vi "Get Pumpstage.vi"(8 "error in (no error)":errorcluster, 11 "VISA resource name":refnum<visa-resource-name>) -> (0 "error out":errorcluster, 1 "Pumpstage (out)":u8, 3 "VISA resource name out":refnum<visa-resource-name>)   [LabVIEW 2018, in "JULABO DeviceDriver.lvlib"]
doc: "This VI returns the acually adjusted pump stage.\n\nNote:\nThis function is not available for uniti which do not support changing the pumpstage. Refer to the units operating manual."
uses:
  JULABO DeviceDriver.lvlib
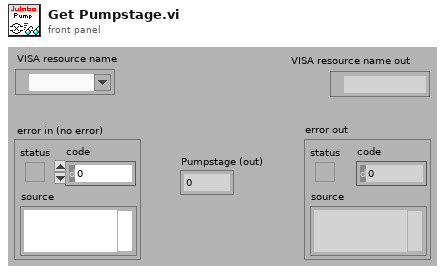
[diagram p1: front panel]
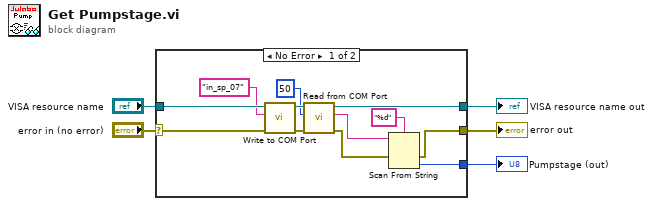
[diagram p0: block diagram]
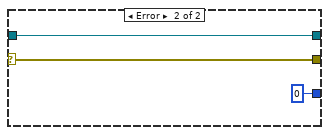
[diagram p2: hidden frame]
diagram:
  n1 = case shown="No Error" "error in (no error)" {
    selector: "error in (no error)" -> [w16 w19]
    tunnel: "VISA resource name" -> [w17 w20]
    tunnel: [w15 w19] -> w3
    tunnel: [w14 w20] -> w2
    tunnel: [w6 0] -> w1
    frame No Error {
      n2 = call "Write to COM Port.vi"("error in"=w16, "Command (input)"="in_sp_07", "VISA resource name in"=w17) -> ("error out"=w13:errorcluster, "VISA resource name out"=w12:refnum<visa-resource-name>)  [unwired: 7 in]
      n3 = call "Read from COM Port.vi"("error in"=w13, "Byte to Read (-1:All)"=u32 50 ("Anzahl der Byte"), "VISA resource name in"=w12) -> ("error out"=w10:errorcluster, "String (output)"=w9:string, "VISA resource name out"=w14:refnum<visa-resource-name>)  [unwired: 5 in, 1 out]
      n4 = Scan From String(format string="%d" ("Format-String"), input string=w9, error in=w10) -> (error out=w15:errorcluster, output 1=w6:i32)  [unwired: 2 in, 2 out]
    }
    frame Error {
    }
  }
  "error out" <- w3
  "VISA resource name out" <- w2
  "Pumpstage (out)" <- w1
